vi "LINX - Analog Read 1 Channel.vi"() -> ()   [LabVIEW 2020]
doc: "Read one the value of one analog channel from a LINX device."
uses:
  vi.lib/MakerHub/LINX/Public/Peripherals/Analog/Analog Read 1 Chan.vi
  vi.lib/MakerHub/LINX/Public/Peripherals/Analog/Analog Read N Chans.vi
  vi.lib/MakerHub/LINX/Private/Local IO/LinxAnalogRead.vi
  vi.lib/MakerHub/LINX/Public/Utilities/Check Channel.vi
  vi.lib/MakerHub/LINX/Public/Utilities/Open Serial.vi
  vi.lib/MakerHub/LINX/Private/Utilties/Generate Error.vi
  vi.lib/MakerHub/LINX/LMH-LINX.lvlib
  vi.lib/MakerHub/LINX/Private/Device/Device.lvlib
panel:
  in  "AI Channel":u8
  out "Loop Rate (Hz)":u32
  in  "Stop Button":bool
  out "Analog Data":dbl(graph)
  in  "Serial Port":refnum<visa-resource-name>
  # "LINX Device Settings"
  # "Analog Value"
  # "Analog Read Example (Serial Interface)\n\nThis example demonstrates how to read analog input values from a LINX device connected to the host computer via Serial / USB.\n\nInstructions\n1. Select the COM Port associated with the LINX Device.\n2. Select the Analog Channel to read.\n3. Click the Run Arrow."
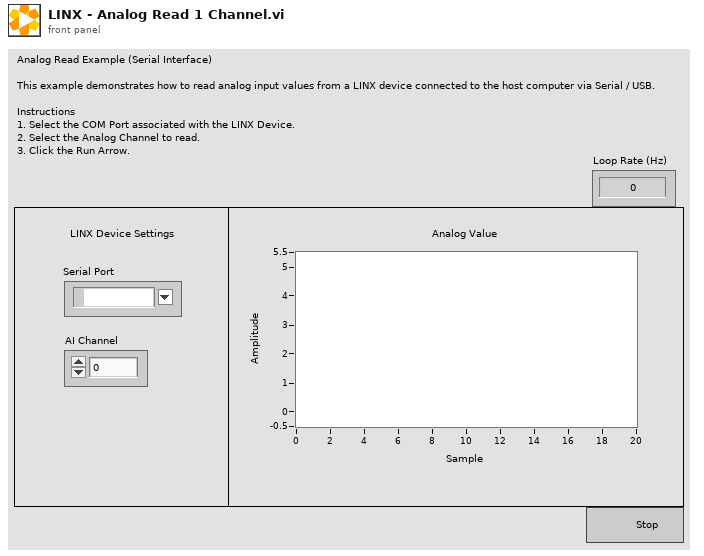
[diagram p1: front panel]
types:
  T1 = typedef "LMH-LINX.lvlib/LINX Ref.ctl" = cluster{"IO":T2, "Interface":T3, "LINX Device Config":T4}
  T2 = typedef "LMH-LINX.lvlib/Platform.ctl" = enum16{"Remote", "Local"}
  T3 = typedef "LMH-LINX.lvlib/Interface.ctl" = enum16{"Serial", "TCP"}
  T4 = typedef "Device.lvlib/LINX Device Config.ctl" = cluster{"Interface":T3, "COM Port":refnum<visa-resource-name>, "TCP Configuration":T5, "Device Family":u8, "Device ID":u8, "Device Name":string, "TCP Ref":refnum<k5>, "Channels":T6}
  T5 = typedef "Device.lvlib/TCP Config.ctl" = cluster{"IP Address":string, "Port":u16}
  T6 = typedef "LMH-LINX.lvlib/Channels.ctl" = cluster{"DI":u8[], "DO":u8[], "AI":u8[], "AO":u8[], "PWM":u8[], "QE":u8[], "UART":u8[], "I2C 2":u8[], "SPI":u8[], "CAN":u8[], "Servo":u8[], "AI Ref (V)":dbl, "AI Resolution (Bits)":u8, "AO Ref (V)":dbl, "AO Resolution (Bits)":u8}
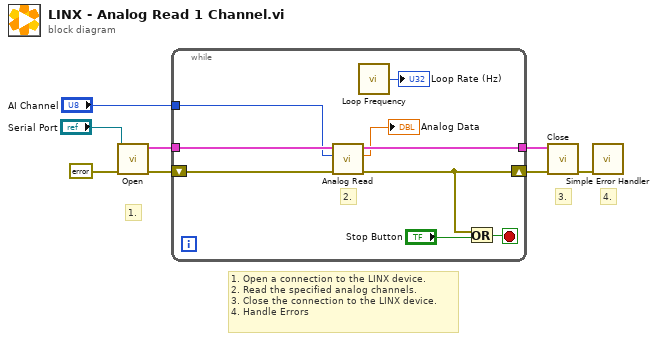
[diagram p0: block diagram]
diagram:
  # "1. Open a connection to the LINX device.\n2. Read the specified analog channels.\n3. Close the connection to the LINX device.\n4. Handle Errors"
  # "4."
  # "3."
  # "1."
  n1 = call-poly "Open.vi"("Error In"=errorcluster {"status"=FALSE, "code"=0, "source"=""}, "Serial Port"="Serial Port") -> ("Error Out"=w7:errorcluster, "LINX Resource"=w8:T1)  [unwired: 7 in, 1 out]
  n2 = while {
    tunnel: w8 -> [w17]
    tunnel: [w15] -> w6
    shift-right: [w12] -> w5
    shift-left: w7 -> [w16]
    tunnel: "AI Channel" -> [w10]
    stop <- w14 stop-if-true
    # "2."
    n3 = call-poly "Analog Read.vi"("Error In"=w16, "Analog Channel"=w10, "LINX Resource"=w17) -> ("Error Out"=w12:errorcluster, "Voltage"=→"Analog Data":dbl, "LINX Resource"=w15:T1)  [unwired: 5 in, 1 out]
    n4 = call "Loop Frequency.vi"() -> ("Loop Rate (Hz)"=→"Loop Rate (Hz)":u32)
    n5 = Or(x=w12, y="Stop Button") -> (x .or. y?=w14:bool)
  }
  n6 = call "Close.vi"("Error In"=w5, "LINX Resource"=w6) -> ("Error Out"=w3:errorcluster)  [unwired: 9 in]
  n7 = call <vilib>:"Simple Error Handler.vi"("error in (no error)"=w3) -> ()  [unwired: 4 in, 5 out]
